vi "SrvDestroy.vi"(0 "ref in":u64, 11 "error in (no error)":errorcluster) -> (15 "error out":errorcluster)   [LabVIEW 2018, in "Snap7.lvlib"]
uses:
  Snap7.lvlib
  windows/lv_snap7.dll
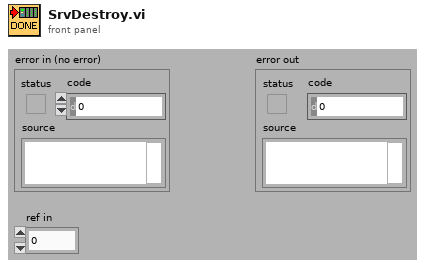
[diagram p1: front panel]
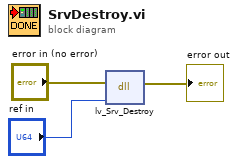
[diagram p0: block diagram]
diagram:
  n1 = dll-call lib="C:/Users/WanLiMing/Downloads/snap7-full-1.4.2/snap7-full-1.4.2/LabVIEW/lib/windows/lv_snap7.dll" fn="lv_Srv_Destroy"(error in="error in (no error)", "Server"="ref in") -> (error out=→"error out":errorcluster)  [unwired: 4 in, 1 out]
